vi "Knock Settings Write.vi"(8 "error in":errorcluster, 9 "Device Inputs":dbl[](array[numeric]), 10 "DCM Ref":refnum<class "DCM - RT.lvclass">, 11 "Knock in":T1={"Knock Enabled"=FALSE, "FIFO Indexes"={"Read"={"Knock"=[-1, -1, -1, -1, -1, -1, -1, -1, -1, -1, -1, -1, -1, -1, -1, -1], "Knock Intensity"=[-1, -1, -1, -1, -1, -1, -1, -1, -1, -1, -1, -1, -1, -1, -1, -1]}, "Write"={"Low Cutoff [Hz]"=-1, "High Cutoff [Hz]"=-1, "Threshold"=-1, "Knock Start [CAD]"=-1, "Knock End [CAD]"=-1, "Reference Start [CAD]"=-1, "Reference End [CAD]"=-1}}, "Settings"={"Sensor Select"=[0, 0, 0, 0, 0, 0, 0, 0, 0, 0, 0, 0, 0, 0, 0, 0], "Cylinder Offset [CAD]"=[0.0, 0.0, 0.0, 0.0, 0.0, 0.0, 0.0, 0.0, 0.0, 0.0, 0.0, 0.0, 0.0, 0.0, 0.0, 0.0]}} {"Settings"."Sensor Select" items=["Sensor 1", "Sensor 2", "Sensor 3", "Sensor 4", "Sensor 5", "Sensor 6", "Sensor 7", "Sensor 8", "Sensor 9", "Sensor 10", "Sensor 11", "Sensor 12"]}) -> (0 "error out":errorcluster)   [LabVIEW 2016, in "DCM Engine.lvlib"]
uses:
  DCM Engine.lvlib
  Built/DCM Classes Packed/Pharlap/C/DCM-Classes.lvlibp/DCM/Rev0/RT/DCM - RT.lvclass
  Shared/Types/Knock.ctl
  Built/DCM Classes Packed/Pharlap/C/DCM-Classes.lvlibp/DCM/Tools/RT/DCM - RT - Tools.lvlib
  DCM Shared.lvlib
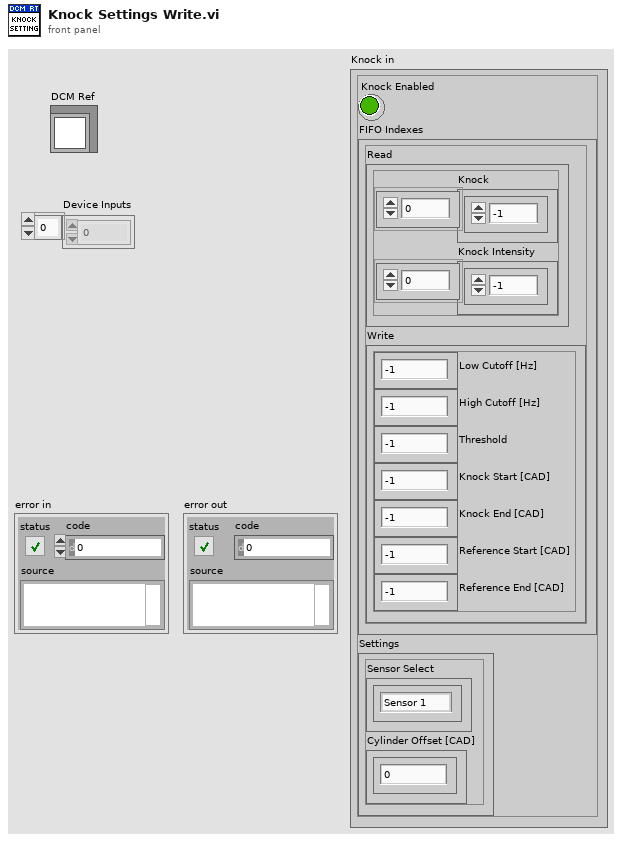
[diagram p1: front panel]
types:
  T1 = typedef "DCM Shared.lvlib/Knock.ctl" = cluster{"Knock Enabled":bool, "FIFO Indexes":cluster{"Read":cluster{"Knock":i32[], "Knock Intensity":i32[]}, "Write":cluster{"Low Cutoff [Hz]":i32, "High Cutoff [Hz]":i32, "Threshold":i32, "Knock Start [CAD]":i32, "Knock End [CAD]":i32, "Reference Start [CAD]":i32, "Reference End [CAD]":i32}}, "Settings":cluster{"Sensor Select":i32[], "Cylinder Offset [CAD]":sgl[]}}
  T2 = cluster{"Low Cutoff [Hz]":i32, "High Cutoff [Hz]":i32, "Threshold":i32, "Knock Start [CAD]":i32, "Knock End [CAD]":i32, "Reference Start [CAD]":i32, "Reference End [CAD]":i32}
  T3 = cluster{"Sensor Select":i32[], "Cylinder Offset [CAD]":sgl[]}
  T4 = typedef "DCM-Classes.lvlibp/DCM - RT - Tools.lvlib/Knock Settings.ctl" = cluster{"Low Cutoff [Hz]":sgl, "High Cutoff [Hz]":sgl, "Threshold":sgl}
  T5 = typedef "DCM-Classes.lvlibp/Knock - RevA - RT.lvlib/Windows.ctl" = cluster{"Knock Start [CAD]":sgl, "Knock End [CAD]":sgl, "Reference Start [CAD]":sgl, "Reference End [CAD]":sgl}
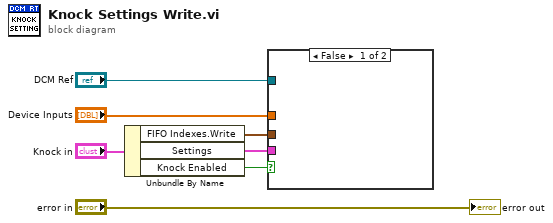
[diagram p0: block diagram]
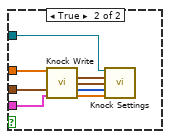
[diagram p2: hidden frame]
diagram:
  n1 = Unbundle By Name("Knock in") -> ("FIFO Indexes.Write"=w2:T2, "Settings"=w3:T3, "Knock Enabled"=w1:bool)
  n2 = case shown="False" w1 {
    tunnel: "DCM Ref" -> [_ w15]
    tunnel: "Device Inputs" -> [_ w14]
    tunnel: w3 -> [_ w9]
    tunnel: w2 -> [_ w8]
    frame False {
    }
    frame True {
      n3 = call "Knock Write.vi"("Device Inputs"=w14, "Controls"=w8, "Settings"=w9) -> ("Knock Settings"=w13:T4, "Knock Windows"=w12:T5, "Knock Sensor"=w11:i32[], "Knock Offset [CAD]"=w10:sgl[])  [unwired: 9 in]
      n4 = call "Knock Settings.vi"("DCM Reference"=w15, "Knock Settings"=w13, "Knock Windows"=w12, "Knock Sensor"=w11, "Knock Offset [CAD]"=w10) -> ()  [unwired: 11 in]
    }
  }
  "error out" <- "error in"
